vi "Immediate Field Centric.vi"(0 "X Setpoint":dbl, 1 "Description":string, 5 "Y Setpoint":dbl, 9 "POV":i16, 11 "Command Info In":T1, 12 "Z Setpoint":dbl, 14 "Gyro":dbl) -> (15 "Command Info Out":T1)   [LabVIEW 2018]
doc: "Often used for joystick control, this VI checks to see that the joystick axes are outside the deadband and updates the motors appropriately."
uses:
  <vilib>/Rock Robotics/WPI/Framework/Command Status Info.ctl
  <vilib>/Rock Robotics/WPI/Framework/Completion Status.ctl
  <vilib>/Rock Robotics/WPI/Framework/Completion Notifier.ctl
  Implementation/Drive Setpoints.ctl
  Implementation/Drive Operations.ctl
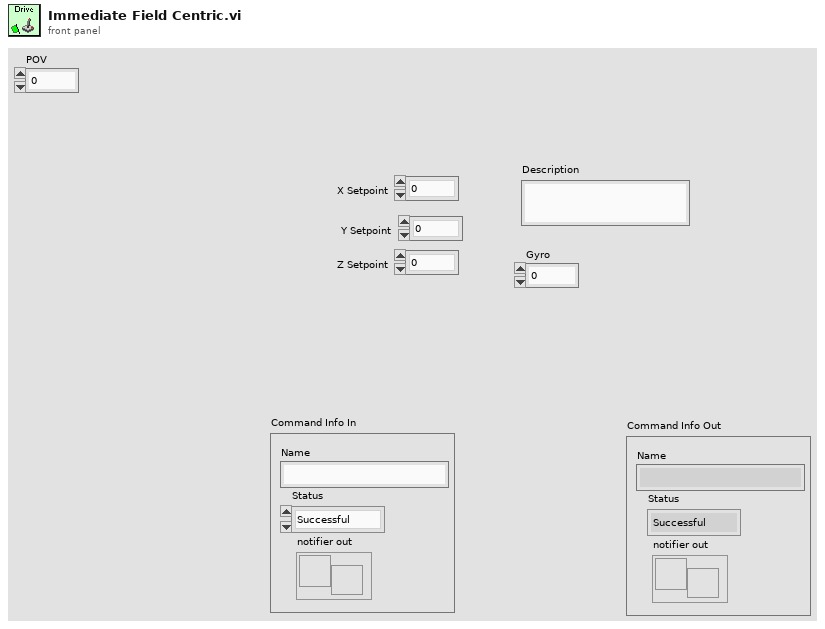
[diagram p1: front panel]
types:
  T1 = typedef "Command Status Info.ctl" = cluster{"Name":string, "Status":T2, "notifier out":T3}
  T2 = typedef "Completion Status.ctl" = enum16{"Successful", "Aborted", "Incomplete"}
  T3 = typedef "Completion Notifier.ctl" = refnum<notifier>
  T4 = typedef "Drive Setpoints.ctl" = cluster{"Operation":T5, "X Setpoint":dbl, "Y Setpoint":dbl, "Duration":dbl, "Z Setpoint":dbl, "Tracks":bool, "Gyro":dbl, "POV":i16, "Distance(feet)":dbl, "AutoTrack Toggle":bool, "Collsision Detection":bool, "Reset Encoder":bool, "MP File Name":string}
  T5 = typedef "Drive Operations.ctl" = enum16{"Reserve", "Read Current", "Reset Motors VBus", "Motion Profile run", "Immediate Robot Centric", "Drive for Time Robot Centric", "Immediate Field Centric", "Drive For Time Field Centric", "Button Adjust", "Set Motors Motion Profile", "Reset Encoders", "Motion Profile Enable", "Drive for Distance"}
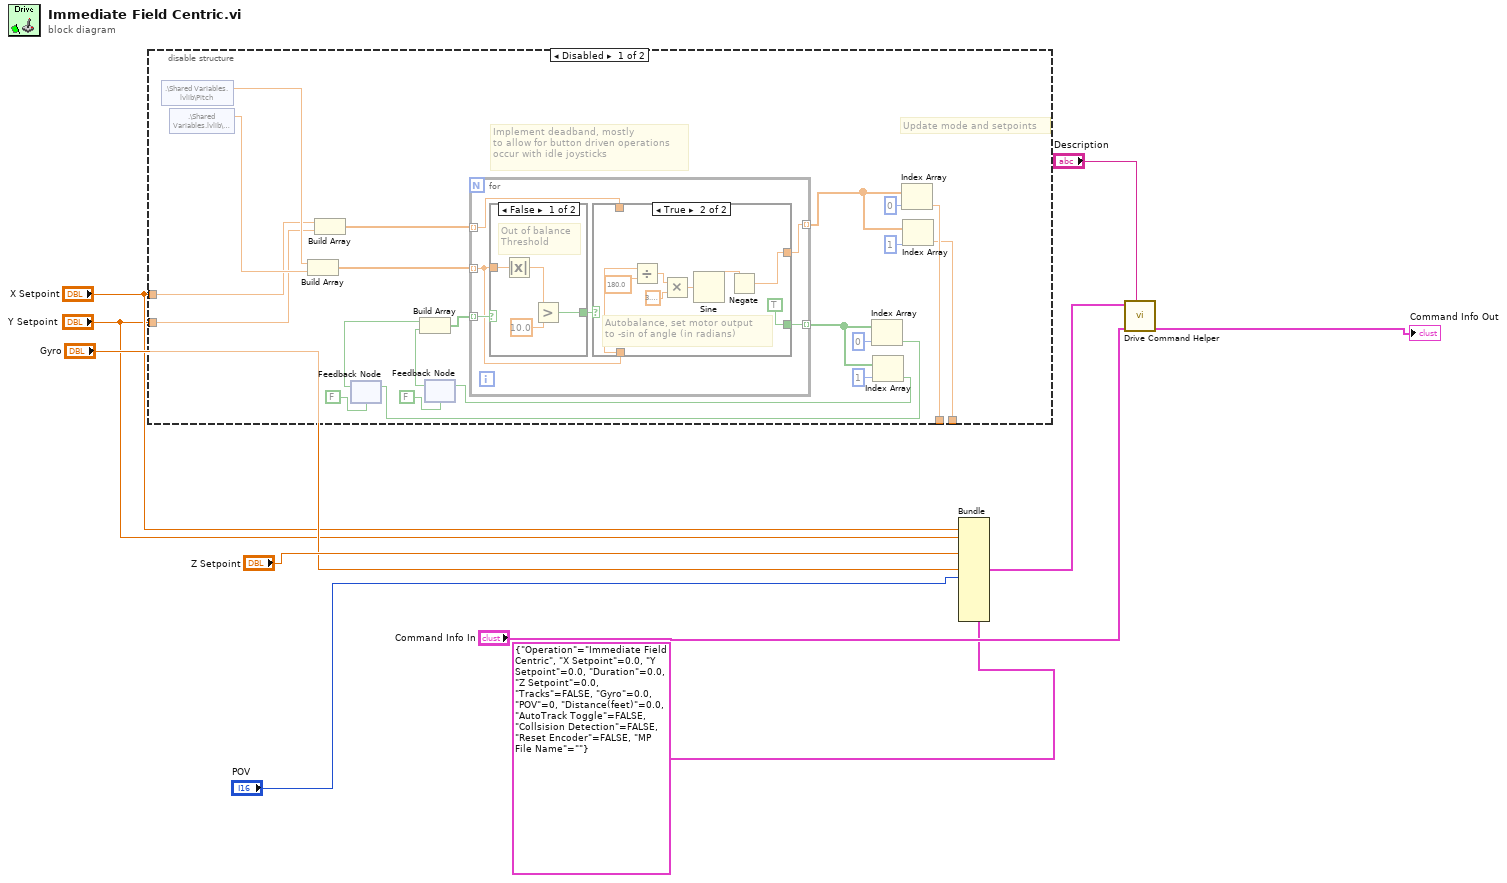
[diagram p0: block diagram]
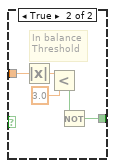
[diagram p2: hidden frame]
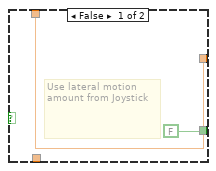
[diagram p3: hidden frame]
diagram:
  n1 = disable-structure shown="Disabled" {
    disable-tunnel: "X Setpoint" -> [w27 _]
    disable-tunnel: "Y Setpoint" -> [w26 _]
    disable-tunnel: [w22 _] -> _
    disable-tunnel: [w21 _] -> _
    frame Disabled {
      # "Implement deadband, mostly\nto allow for button driven operations\noccur with idle joysticks"
      # "Update mode and setpoints"
      n2 = shared-variable ".\\Shared Variables.lvlib\\Pitch"() -> (w30:dbl)  [unwired: 1 in, 1 out]
      n3 = shared-variable ".\\Shared Variables.lvlib\\Roll"() -> (w29:dbl)  [unwired: 1 in, 1 out]
      n4 = Build Array(w30, w29) -> (w31:dbl[])
      n5 = Build Array(w27, w26) -> (w28:dbl[])
      n6 = feedback #1(FALSE) -> (w15:bool)
      n7 = feedback #2(FALSE) -> (w14:bool)
      n8 = Build Array(w15, w14) -> (w13:bool[])
      n9 = for {
        tunnel: w13 -> [w36] mode=indexing
        tunnel: w28 -> [w32] mode=indexing
        tunnel: [w35] -> w18 mode=indexing
        tunnel: [w34] -> w23 mode=indexing
        tunnel: w31 -> [w33] mode=indexing
        n10 = case shown="False" w36 {
          tunnel: w33 -> [w41 w44]
          tunnel: [w38 w43] -> w37
          frame False {
            # "Out of balance\nThreshold"
            n11 = Absolute Value(x=w41) -> (abs(x)=w40:dbl)
            n12 = Greater?(x=w40, y=10.0) -> (0:w38:bool)
          }
          frame True {
            # "In balance\nThreshold"
            n13 = Absolute Value(x=w44) -> (abs(x)=w45:dbl)
            n14 = Less?(x=w45, y=3.0) -> (x < y?=w42:bool)
            n15 = Not(x=w42) -> (.not. x?=w43:bool)
          }
        }
        n16 = case shown="True" w37 {
          tunnel: w33 -> [_ w55]
          tunnel: [w47 w49] -> w34
          tunnel: [FALSE TRUE] -> w35
          tunnel: w32 -> [w47 _]
          frame False {
            # "Use lateral motion amount from Joystick"
          }
          frame True {
            # "Autobalance, set motor output \nto -sin of angle (in radians)"
            n17 = Divide(x=w55, y=180.0) -> (x/y=w53:dbl)
            n18 = Multiply(x=w53, y=3.141592653589793) -> (x*y=w51:dbl)
            n19 = Sine(x=w51) -> (sin(x)=w50:dbl)
            n20 = Negate(x=w50) -> (-x=w49:dbl)
          }
        }
      }
      n21 = Index Array(array=w18, index=0) -> (element=w11:bool)
      n22 = feedback-in #1(w11) -> ()
      n23 = Index Array(array=w18, index=1) -> (element=w12:bool)
      n24 = feedback-in #2(w12) -> ()
      n25 = Index Array(array=w23, index=0) -> (element=w22:dbl)
      n26 = Index Array(array=w23, index=1) -> (element=w21:dbl)
    }
    frame Enabled {
    }
  }
  n27 = Bundle(cluster=T4 {"Operation"=enum."Immediate Field Centric", "X Setpoint"=0.0, "Y Setpoint"=0.0, "Duration"=0.0, "Z Setpoint"=0.0, "Tracks"=FALSE, "Gyro"=0.0, "POV"=0, "Distance(feet)"=0.0, "AutoTrack Toggle"=FALSE, "Collsision Detection"=FALSE, "Reset Encoder"=FALSE, "MP File Name"=""} ("SubSystem Data"), "X Setpoint"="X Setpoint", "Y Setpoint"="Y Setpoint", "Z Setpoint"="Z Setpoint", "Gyro"="Gyro", "POV"="POV") -> (w4:T4)  [unwired: 8 in]
  n28 = call "Drive Command Helper.vi"("Description"="Description", "Command Info In"="Command Info In", "SubSystem Data"=w4) -> ("Command Info Out"=→"Command Info Out":T1)  [unwired: 7 in, 1 out]
